vi "test Deployment Disabled Custom Device.vi"(8 "error in":errorcluster, 11 "reference in":refnum<class "AIM ARINC 664 Deployment.lvclass">) -> (0 "error out":errorcluster, 3 "reference out":refnum<class "AIM ARINC 664 Deployment.lvclass">)   [LabVIEW 2020, in "AIM ARINC 664 Deployment.lvclass"]
uses:
  AIM ARINC 664 Deployment.lvclass
  AIM ARINC 664 Deployment.lvclass/AIM ARINC 664 Deployment.ctl
  1575c155-adf8-4776-b0d3-988305b88d42.vi
  ffd82da4-029b-4353-8800-b1105752ddcc.vi
  <vilib>/NI/VeriStand Custom Device Testing Tools/VeriStandTestUtilities/VeriStandTestUtilities.lvlib
  Scripting/AIM ARINC 664 Scripting.lvlib
  <vilib>/addons/_JKI Toolkits/VI Tester/TestCase.llb/TestCase.lvclass
  C:/Program Files (x86)/National Instruments/LabVIEW 2020/vi.lib/addons/_JKI Toolkits/VI Tester/TestCase.llb/TestCase.lvclass
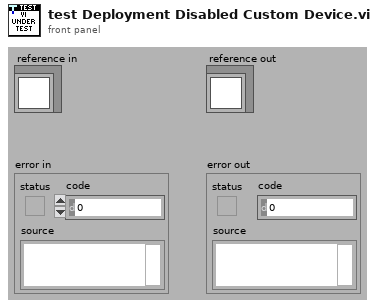
[diagram p1: front panel]
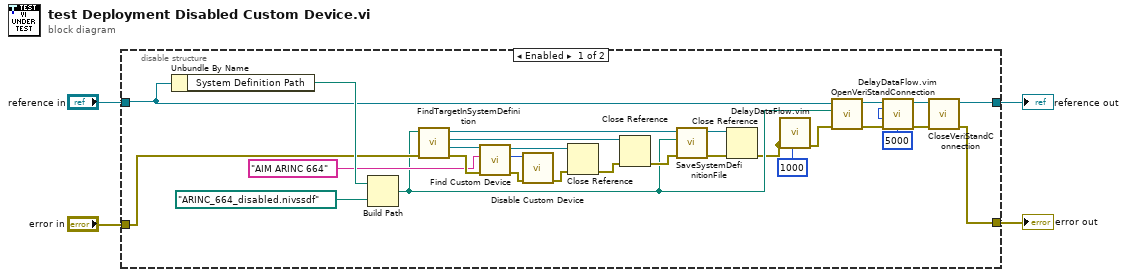
[diagram p0: block diagram]
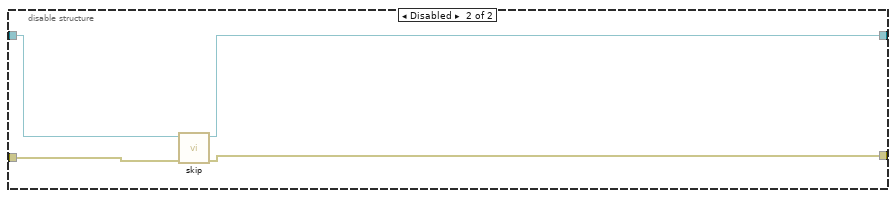
[diagram p2: hidden frame]
diagram:
  n1 = disable-structure shown="Enabled" {
    disable-tunnel: "reference in" -> [w12 w35]
    disable-tunnel: "error in" -> [w11 w34]
    disable-tunnel: [w9 w33] -> w2
    disable-tunnel: [w10 w32] -> w1
    frame Enabled {
      n2 = Unbundle By Name(w12) -> ("System Definition Path"=w25:path)
      n3 = Build Path(base path=w25, name or relative path=path "ARINC_664_disabled.nivssdf") -> (appended path=w8:path)
      n4 = call <vilib>:"FindTargetInSystemDefinition.vi"("error in"=w11, "system definition path"=w8) -> ("error out"=w27:errorcluster, "Target"=w26:refnum<k24>, "Root"=w21:refnum<k24>, "System Definition"=w24:refnum<k24>)  [unwired: 6 in]
      n5 = call "Find Custom Device.vi"("error in"=w27, "name"="AIM ARINC 664" ("custom device name"), "target in"=w26) -> ("error out"=w29:errorcluster, "custom device"=w28:u64, "target out"=w31:refnum<k24>)  [unwired: 6 in]
      n6 = call "Disable Custom Device.vi"("error in"=w29, "custom device ref in"=w28) -> ("error out"=w30:errorcluster)  [unwired: 8 in, 1 out]
      n7 = Close Reference(reference=w31, error in (no error)=w30) -> (error out=w19:errorcluster)
      n8 = Close Reference(reference=w21, error in (no error)=w19) -> (error out=w20:errorcluster)
      n9 = call <vilib>:"SaveSystemDefinitionFile.vi"("error in (no error)"=w20, "System Definition File in"=w8, "System Definition Reference in"=w24) -> ("error out"=w22:errorcluster, "System Definition Reference out"=w23:refnum<k24>)  [unwired: 7 in]
      n10 = Close Reference(reference=w23, error in (no error)=w22) -> (error out=w6:errorcluster)
      n11 = call "DelayDataFlow.vim"("value in"=w6, "milliseconds to wait"=u32 1000, "no delay on error (T)"=w6) -> ("value out"=w5:errorcluster)  [unwired: 1 in, 1 out]
      n12 = call-dynamic "OpenVeriStandConnection.vi"("error in (no error)"=w5, "System Definition File"=w8, "VeriStand Test Case in"=w12) -> ("error out"=w16:errorcluster, "VeriStand Test Case out"=w18:refnum<class "AIM ARINC 664 Deployment.lvclass">)  [unwired: 6 in, 1 out]
      n13 = call "DelayDataFlow.vim"("value in"=w16, "milliseconds to wait"=u32 5000) -> ("value out"=w17:errorcluster)  [unwired: 2 in, 1 out]
      n14 = call-dynamic "CloseVeriStandConnection.vi"("error in (no error)"=w17, "VeriStand Test Case in"=w18) -> ("error out"=w9:errorcluster, "VeriStand Test Case out"=w10:refnum<class "AIM ARINC 664 Deployment.lvclass">)  [unwired: 8 in]
    }
    frame Disabled {
      n15 = call <vilib>:"skip.vi"("error in (no error)"=w34, "TestCase in"=w35) -> ("error out"=w33:errorcluster, "TestCase out"=w32:refnum<class "AIM ARINC 664 Deployment.lvclass">)  [unwired: 8 in]
    }
  }
  "error out" <- w2
  "reference out" <- w1
